vi "New.vi"(8 "error in (no error)":errorcluster, 9 "Error/Abort details (JSON)":T1={"Error URI"="", "Error Arguments"="[]", "Error ArgumentKw"="{}", "Error Details"="{}", "Associated LabVIEW Error"={"status"=FALSE, "code"=0, "source"=""}}, 10 "Request URI":string, 11 "Success?":bool=TRUE) -> (0 "error out":errorcluster, 3 "ErrorOrSuccess JSON out":refnum<class "ErrorOrSuccess JSON.lvclass">)   [LabVIEW 2020, in "wamplv.lvlib" / "ErrorOrSuccess JSON.lvclass"]
uses:
  ErrorOrSuccess JSON.lvclass
  WAMP Client/API/TypeDefs/Error or abort detail (JSON).ctl
  ErrorOrSuccess JSON.lvclass/ErrorOrSuccess JSON.ctl
  C:/local/wamplv/Private/Message loop classes/ErrorOrSuccess/ErrorOrSuccess.lvclass
  C:/local/wamplv/Private/Message loop classes/ErrorOrSuccess JSON/ErrorOrSuccess JSON.lvclass
  ErrorOrSuccess/ErrorOrSuccess.lvclass
  wamplv.lvlib
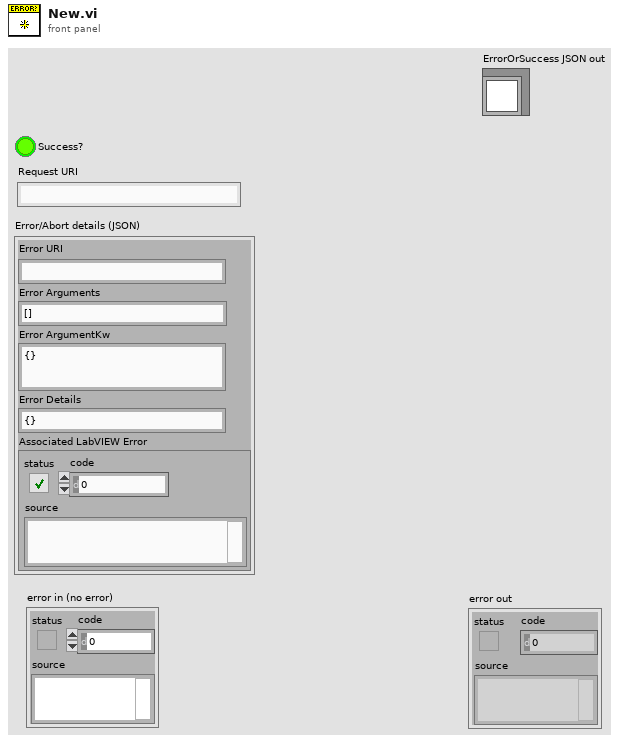
[diagram p1: front panel]
types:
  T1 = typedef "wamplv.lvlib/Error or abort detail (JSON).ctl" = cluster{"Error URI":string, "Error Arguments":string, "Error ArgumentKw":string, "Error Details":string, "Associated LabVIEW Error":errorcluster}
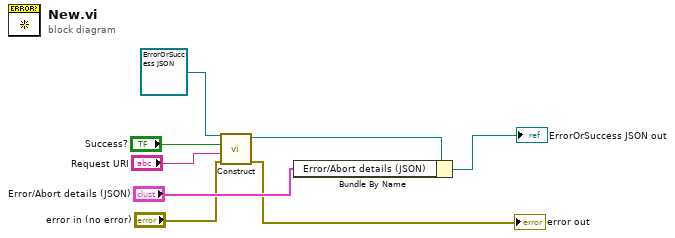
[diagram p0: block diagram]
diagram:
  n1 = call "Construct.vi"("error in (no error)"="error in (no error)", "Request URI"="Request URI", "Success?"="Success?", "ErrorOrSuccess in"=refnum<class "ErrorOrSuccess JSON.lvclass"> refnum ("wamplv.lvlib:ErrorOrSuccess JSON.lvclass")) -> ("error out"=→"error out":errorcluster, "ErrorOrSuccess out"=w5:refnum<class "ErrorOrSuccess JSON.lvclass">)  [unwired: 6 in]
  n2 = Bundle By Name(cluster=w5, "Error/Abort details (JSON)"="Error/Abort details (JSON)") -> (→"ErrorOrSuccess JSON out":refnum<class "ErrorOrSuccess JSON.lvclass">)
